vi "Finalize.vi"(8 "error in":errorcluster, 11 "AIM ARINC-429 logging execution unit in":refnum<class "Logging Execution Unit.lvclass">) -> (0 "error out":errorcluster, 3 "AIM ARINC-429 logging execution unit out":refnum<class "Logging Execution Unit.lvclass">)   [LabVIEW 2020, in "AIM ARINC 429 Engine.lvlib" / "Implementation.lvlib" / "Logging Execution Unit.lvclass"]
uses:
  Logging Execution Unit.lvclass
  C:/Git/niveristand-aim-arinc429-custom-device/Source/Custom Device Support/Engine/Implementation/Execution Unit/Execution Unit.lvclass
  Execution Unit/Execution Unit.lvclass/Execution Unit.ctl
  <instrlib>/AIM GmbH/ARINC-429/subvi/Error Converter (ErrCode or Status).vi
  <instrlib>/AIM GmbH/ARINC-429/subvi/Get Library Path.vi
  <instrlib>/AIM GmbH/ARINC-429/VIs/Library/Api429Lib Error Desc Get.vi
  <instrlib>/AIM GmbH/ARINC-429/subvi/Get Error Number Offset.vi
  <vilib>/Utility/error.llb/Error Cluster From Error Code.vi
  <instrlib>/AIM GmbH/ARINC-429/AIM429LV.lvlib
  Execution Unit/Execution Unit.lvclass
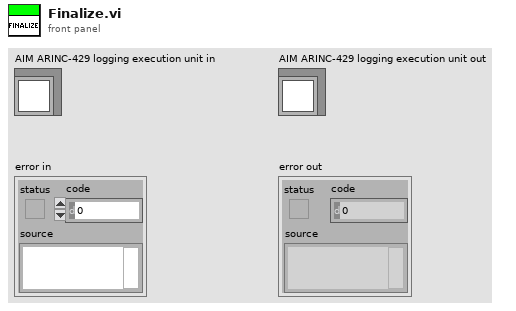
[diagram p1: front panel]
types:
  T1 = typedef "AIM ARINC 429 Engine.lvlib/Custom Device.lvlib/Hardware Handles.ctl" = cluster{"module":u8}
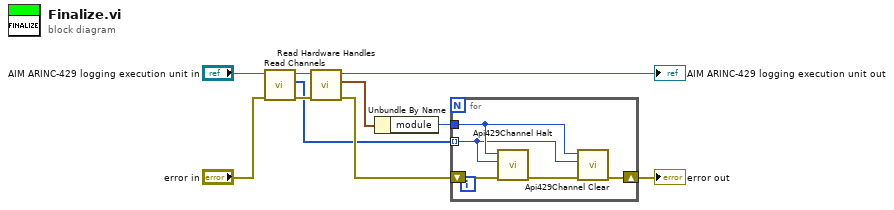
[diagram p0: block diagram]
diagram:
  n1 = call "Read Channels.vi"("error in"="error in", "execution unit in"="AIM ARINC-429 logging execution unit in") -> ("error out"=w3:errorcluster, "channels"=w1:u8[], "execution unit out"=w2:refnum<class "Logging Execution Unit.lvclass">)  [unwired: 7 in]
  n2 = call "Read Hardware Handles.vi"("error in"=w3, "AIM ARINC-429 execution unit in"=w2) -> ("error out"=w9:errorcluster, "hardware handles"=w8:T1, "AIM ARINC-429 execution unit out"=→"AIM ARINC-429 logging execution unit out":refnum<class "Logging Execution Unit.lvclass">)  [unwired: 7 in]
  n3 = Unbundle By Name(w8) -> ("module"=w7:u8)
  n4 = for {
    shift-right: [w13] -> w10
    shift-left: w9 -> [w14]
    tunnel: w1 -> [w11] mode=indexing
    tunnel: w7 -> [w12]
    n5 = call <instrlib>:"Api429Channel Halt.vi"("error in (no error)"=w14, "channel_id"=w11, "board_handle"=w12) -> ("error out"=w15:errorcluster)  [unwired: 8 in]
    n6 = call <instrlib>:"Api429Channel Clear.vi"("error in (no error)"=w15, "channel_id"=w11, "board_handle"=w12) -> ("error out"=w13:errorcluster)  [unwired: 8 in]
  }
  "error out" <- w10
